vi "Ch_setup_string.vi"(5 "Analysis Info cluster (An Chs)":T1[](array[typedef])=[{"Colour"=0, "Inst type"=enum."Pitot-static tube", "Inst name"="Manometer voltage", "Symbol"="U", "Code name"="", "Extra Info"="U", "Inst Array"=enum."PWA", "Index"=0, "Voltage Index"=0, "Extra Titles"=[], "Extra Values"=[]}, {"Colour"=0, "Inst type"=enum."Pitot-static tube", "Inst name"="Manometer voltage", "Symbol"="U", "Code name"="", "Extra Info"="U", "Inst Array"=enum."PWA", "Index"=0, "Voltage Index"=0, "Extra Titles"=[], "Extra Values"=[]}, {"Colour"=0, "Inst type"=enum."Pitot-static tube", "Inst name"="Manometer voltage", "Symbol"="U", "Code name"="", "Extra Info"="U", "Inst Array"=enum."PWA", "Index"=0, "Voltage Index"=0, "Extra Titles"=[], "Extra Values"=[]}, {"Colour"=0, "Inst type"=enum."Pitot-static tube", "Inst name"="Manometer voltage", "Symbol"="U", "Code name"="", "Extra Info"="U", "Inst Array"=enum."PWA", "Index"=0, "Voltage Index"=0, "Extra Titles"=[], "Extra Values"=[]}], 6 "Ch & spans":T4[](array[typedef]) {"low limit (-10V)" format="%.3f"; "high limit (10V)" format="%.3f"}) -> (1 "Output string":string)   [LabVIEW 2010]
uses:
  Controls/Ch_and_Spans.ctl
  Controls/Analysis_info_cluster.ctl
  Controls/Inst_type.ctl
  Controls/Instrument_Array.ctl
  Globals/Meas_global.vi
panel:
  out "length":i32
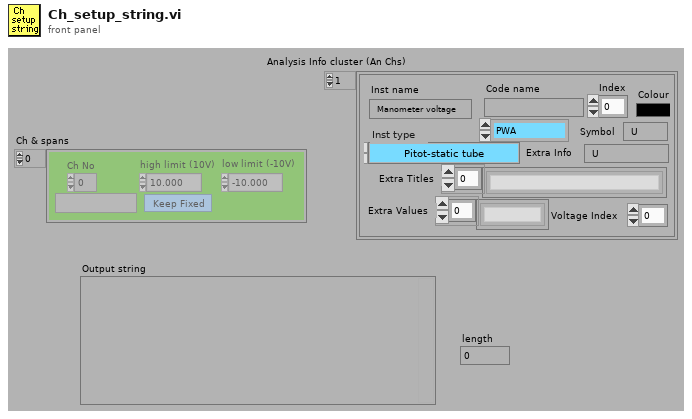
[diagram p1: front panel]
types:
  T1 = typedef "Analysis_info_cluster.ctl" = cluster{"Colour":u32, "Inst type":T2, "Inst name":string, "Symbol":string, "Code name":string, "Extra Info":string, "Inst Array":T3, "Index":i32, "Voltage Index":i32, "Extra Titles":string[], "Extra Values":string[]}
  T2 = typedef "Inst_type.ctl" = enum16{"Propeller anemometer", "Raw voltage", "Pressure Transducer", "Pitot-static tube", "Preston tube", "Hot wire", "Cross wire 1", "Cross wire 2", "Generic Linear", "Generic Polynomial", "Generic BackPoly", "Fast FID", "Thermocouple", "Cold wire", "Pulsed Wire", "LDA Vel", "LDA Tran time", "LDA Arr time"}
  T3 = typedef "Instrument_Array.ctl" = enum16{"PWA", "LDA", "Analogue"}
  T4 = typedef "Ch_and_Spans.ctl" = cluster{"high limit (10V)":sgl, "low limit (-10V)":sgl, "Ch No":i16, "Var name":string, "Use Latest Calib":bool}
  T5 = cluster{"Name":string, "X":dbl, "Y":dbl, "Z":dbl}[]
  T6 = typedef "PWA_Data.ctl" = enum16{"No PWA Data", "One Ch PWA"}
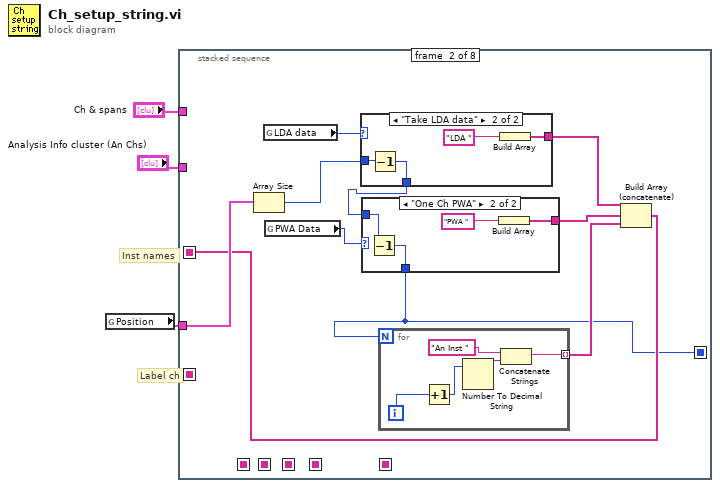
[diagram p0: block diagram]
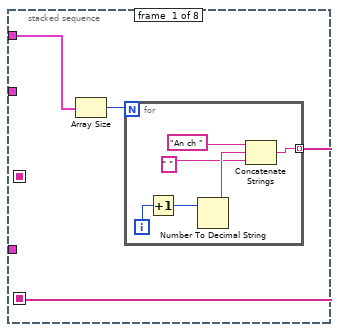
[diagram p2: hidden frame]
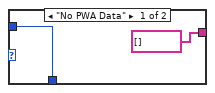
[diagram p3: hidden frame]
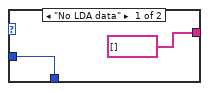
[diagram p4: hidden frame]
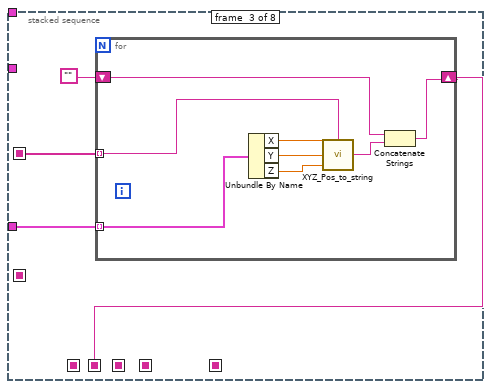
[diagram p5: hidden frame]
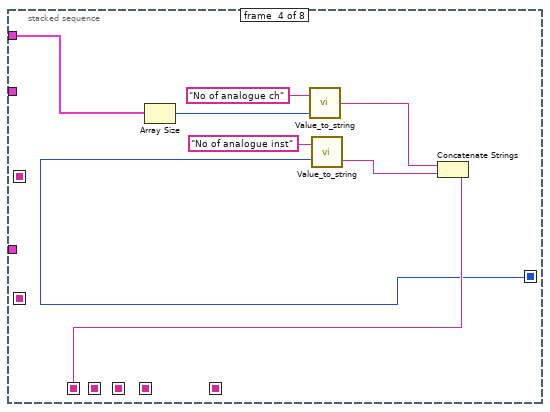
[diagram p6: hidden frame]
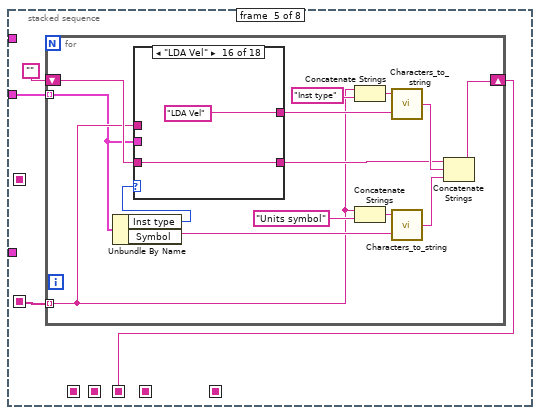
[diagram p7: hidden frame]
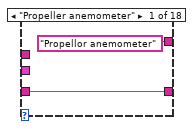
[diagram p8: hidden frame]
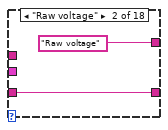
[diagram p9: hidden frame]
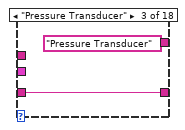
[diagram p10: hidden frame]
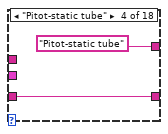
[diagram p11: hidden frame]
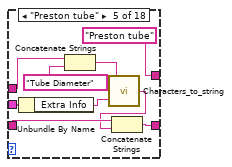
[diagram p12: hidden frame]
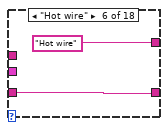
[diagram p13: hidden frame]
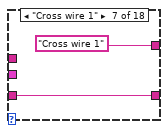
[diagram p14: hidden frame]
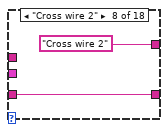
[diagram p15: hidden frame]
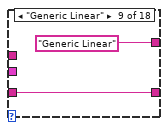
[diagram p16: hidden frame]
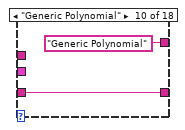
[diagram p17: hidden frame]
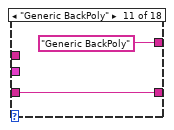
[diagram p18: hidden frame]
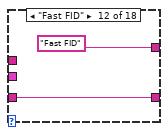
[diagram p19: hidden frame]
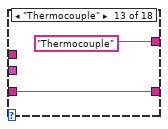
[diagram p20: hidden frame]
diagram:
  # "Inst names"
  # "Label ch"
  n1 = global read "Meas_global.vi" "Position"() -> (w3:T5)
  n2 = stacked-sequence {
    seq-local: [_ _ _ _ w62 _ _ _] -> [_ _ _ _ _ _ _ w166]
    seq-local: [_ _ _ _ _ _ w149 _] -> [_ _ _ _ _ _ _ w165]
    seq-local: [_ _ w42 _ _ _ _ _] -> [_ _ _ _ _ _ _ w164]
    seq-local: [w5 _ _ _ _ _ _ _] -> [_ _ _ _ w61 w123 w150 _]
    seq-local: [_ _ _ w54 _ _ _ _] -> [_ _ _ _ _ _ _ w161]
    seq-local: [_ _ _ _ _ w122 _ _] -> [_ _ _ _ _ _ _ w160]
    seq-local: [_ w14 _ _ _ _ _ _] -> [_ _ _ w53 _ _ _ _]
    seq-local: [_ w17 _ _ _ _ _ _] -> [_ _ w40 _ _ _ _ _]
    tunnel: w3 -> [_ w21 w41 _ _ _ _ _]
    tunnel: "Ch & spans" -> [w4 _ _ w52 _ w121 _ _]
    tunnel: "Analysis Info cluster (An Chs)" -> [_ _ _ _ w60 _ _ _]
    frame #0 {
      n3 = Array Size(array=w4) -> (size(s)=w6:i32)
      n4 = for {
        N: w6 -> [_]
        tunnel: [w8] -> w5 mode=indexing
        i -> [w10]
        n5 = Increment(x=w10) -> (x+1=w9:i32)
        n6 = Number To Decimal String(number=w9) -> (decimal integer string=w12:string)  [unwired: 1 out]
        n7 = Concatenate Strings("An ch ", w12, " ") -> (w8:string)
      }
    }
    frame #1 {
      n8 = Array Size(array=w21) -> (size(s)=w20:i32)
      n9 = global read "Meas_global.vi" "LDA data"() -> (w22:enum16{"No LDA data", "Take LDA data"})
      n10 = global read "Meas_global.vi" "PWA Data"() -> (w16:T6)
      n11 = case shown="\"Take LDA data\"" w22 {
        tunnel: [w35 w38] -> w15
        tunnel: w20 -> [w35 w39]
        tunnel: [string[] [] w36] -> w19
        frame "No LDA data" {
        }
        frame "Take LDA data" {
          n12 = Decrement(x=w39) -> (x-1=w38:i32)
          n13 = Build Array("LDA ") -> (w36:string[])
        }
      }
      n14 = case shown="\"One Ch PWA\"" w16 {
        tunnel: [w24 w27] -> w14
        tunnel: w15 -> [w24 w28]
        tunnel: [string[] [] w25] -> w13
        frame "No PWA Data" {
        }
        frame "One Ch PWA" {
          n15 = Decrement(x=w28) -> (x-1=w27:i32)
          n16 = Build Array("PWA ") -> (w25:string[])
        }
      }
      n17 = for {
        N: w14 -> [_]
        tunnel: [w29] -> w18 mode=indexing
        i -> [w30]
        n18 = Increment(x=w30) -> (x+1=w31:i32)
        n19 = Number To Decimal String(number=w31) -> (decimal integer string=w33:string)  [unwired: 1 out]
        n20 = Concatenate Strings("An Inst ", w33) -> (w29:string)
      }
      n21 = Build Array (concatenate)(w19, w13, w18) -> (w17:string[])
    }
    frame #2 {
      n22 = for {
        shift-right: [w50] -> w42
        shift-left: "" -> [w51]
        tunnel: w41 -> [w49] mode=indexing
        tunnel: w40 -> [w44] mode=indexing
        n23 = Unbundle By Name(w49) -> ("X"=w46:dbl, "Y"=w47:dbl, "Z"=w48:dbl)
        n24 = call "XYZ_Pos_to_string.vi"("Position label"=w44, "Z"=w48, "Y"=w47, "X"=w46) -> ("Output string"=w45:string)
        n25 = Concatenate Strings(w51, w45) -> (w50:string)
      }
    }
    frame #3 {
      n26 = Array Size(array=w52) -> (size(s)=w57:i32)
      n27 = call "Value_to_string.vi"("Value"=w57, "Label for value"="No of analogue ch") -> ("Output string"=w56:string)  [unwired: 1 in]
      n28 = call "Value_to_string.vi"("Value"=w53, "Label for value"="No of analogue inst") -> ("Output string"=w55:string)  [unwired: 1 in]
      n29 = Concatenate Strings(w56, w55) -> (w54:string)
    }
    frame #4 {
      n30 = for {
        shift-right: [w77] -> w62
        shift-left: "" -> [w68]
        tunnel: w61 -> [w65] mode=indexing
        tunnel: w60 -> [w64] mode=indexing
        n31 = Unbundle By Name(w64) -> ("Inst type"=w66:T2, "Symbol"=w76:string)
        n32 = case shown="\"LDA Vel\"" w66 {
          tunnel: ["Propellor anemometer" "Raw voltage" "Pressure Transducer" "Pitot-static tube" "Preston tube" "Hot wire" "Cross wire 1" "Cross wire 2" "Generic Linear" "Generic Polynomial" "Generic BackPoly" "Fast FID" "Thermocouple" "Cold wire" "Pulsed wire" "LDA Vel" "LDA Tran time" "LDA Arr time"] -> w75
          tunnel: w68 -> [w78 w80 w82 w84 w92 w95 w97 w99 w101 w103 w105 w107 w109 w111 w113 w115 w117 w119]
          tunnel: [w78 w80 w82 w84 w91 w95 w97 w99 w101 w103 w105 w107 w109 w111 w113 w115 w117 w119] -> w67
          tunnel: w64 -> [_ _ _ _ w94 _ _ _ _ _ _ _ _ _ _ _ _ _]
          tunnel: w65 -> [_ _ _ _ w87 _ _ _ _ _ _ _ _ _ _ _ _ _]
          frame "Propeller anemometer" {
          }
          frame "Raw voltage" {
          }
          frame "Pressure Transducer" {
          }
          frame "Pitot-static tube" {
          }
          frame "Preston tube" {
            n33 = Unbundle By Name(w94) -> ("Extra Info"=w93:string)
            n34 = Concatenate Strings(w87, "Tube Diameter") -> (w86:string)
            n35 = call "Characters_to_string.vi"("Characters to write"=w93, "Label for characters"=w86) -> ("Output string"=w89:string)
            n36 = Concatenate Strings(w92, w89) -> (w91:string)
          }
          frame "Hot wire" {
          }
          frame "Cross wire 1" {
          }
          frame "Cross wire 2" {
          }
          frame "Generic Linear" {
          }
          frame "Generic Polynomial" {
          }
          frame "Generic BackPoly" {
          }
          frame "Fast FID" {
          }
          frame "Thermocouple" {
          }
          frame "Cold wire" {
          }
          frame "Pulsed Wire" {
          }
          frame "LDA Vel" {
          }
          frame "LDA Tran time" {
          }
          frame "LDA Arr time" {
          }
        }
        n37 = Concatenate Strings(w65, "Inst type") -> (w69:string)
        n38 = Concatenate Strings(w65, "Units symbol") -> (w70:string)
        n39 = call "Characters_to_string.vi"("Characters to write"=w75, "Label for characters"=w69) -> ("Output string"=w71:string)
        n40 = call "Characters_to_string.vi"("Characters to write"=w76, "Label for characters"=w70) -> ("Output string"=w72:string)
        n41 = Concatenate Strings(w67, w71, w72) -> (w77:string)
      }
    }
    frame #5 {
      n42 = for {
        shift-right: [w146] -> w122
        shift-left: "" -> [w147]
        tunnel: w123 -> [w133] mode=indexing
        tunnel: w121 -> [w127] mode=indexing
        n43 = Unbundle By Name(w127) -> ("high limit (10V)"=w134:sgl, "low limit (-10V)"=w135:sgl, "Ch No"=w136:i16, "Use Latest Calib"=w126:bool)
        n44 = Select(t="TRUE", s=w126, f="FALSE") -> (s? t:f=w128:string)
        n45 = Concatenate Strings(w133, "Use latest Calib") -> (w131:string)
        n46 = Concatenate Strings(w133, "High limit") -> (w143:string)
        n47 = Concatenate Strings(w133, "Low limit") -> (w142:string)
        n48 = Concatenate Strings(w133, "Ch No") -> (w139:string)
        n49 = call "Value_to_string.vi"("Value"=w134, "Label for value"=w143) -> ("Output string"=w144:string)  [unwired: 1 in]
        n50 = call "Value_to_string.vi"("Value"=w135, "Label for value"=w142) -> ("Output string"=w138:string)  [unwired: 1 in]
        n51 = call "Value_to_string.vi"("Value"=w136, "Label for value"=w139) -> ("Output string"=w137:string)  [unwired: 1 in]
        n52 = call "Characters_to_string.vi"("Characters to write"=w128, "Label for characters"=w131) -> ("Output string"=w125:string)
        n53 = Concatenate Strings(w147, w144, w138, w137, w125) -> (w146:string)
      }
    }
    frame #6 {
      n54 = global read "Meas_global.vi" "Calib files"() -> (w148:path[])
      n55 = for {
        shift-right: [w158] -> w149
        shift-left: "" -> [w159]
        tunnel: w150 -> [w154] mode=indexing
        tunnel: w148 -> [w152] mode=indexing
        n56 = Path To String(path=w152) -> (string=w153:string)
        n57 = Concatenate Strings(w154, "Calib filename") -> (w155:string)
        n58 = call "Characters_to_string.vi"("Characters to write"=w153, "Label for characters"=w155) -> ("Output string"=w156:string)
        n59 = Concatenate Strings(w159, w156) -> (w158:string)
      }
    }
    frame #7 {
      n60 = Concatenate Strings(w161, w164, w166, w165, w160) -> (w162:string)
      "Output string" <- w162
      n61 = String Length(string=w162) -> (length=→"length":i32)
    }
  }
